vi "Scan Project Items.vi"(6 "Slide in":refnum<vi>, 7 "Project Path":path, 8 "error in (no error)":errorcluster, 10 "VI Refnum":refnum<vi>, 11 "Member Data in":string[][](array[string])) -> (0 "error out":errorcluster, 3 "Member Data out":string[][](array[string]))   [LabVIEW 2014]
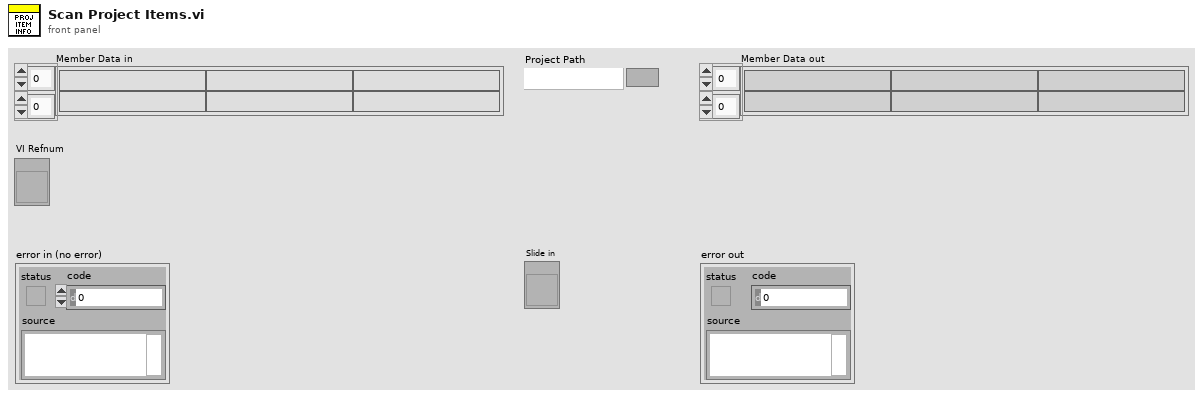
[diagram p1: front panel]
types:
  T1 = typedef "TYPE_Description Cluster.ctl" = cluster{"VI Description":string, "VI Version":string, "Review Date":string, "Author":string, "Copyright":string, "Requirements Coverage":string}
  T2 = typedef "TYPE_Version Status.ctl" = enum16{"Development", "alpha", "beta", "Reviewed", "Bug", "Other"}
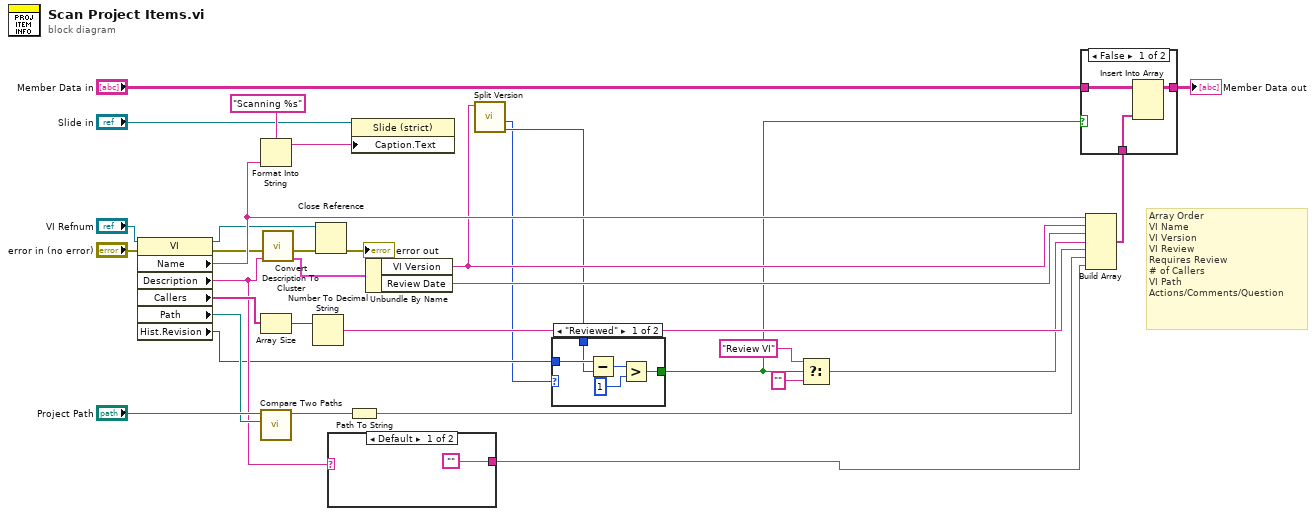
[diagram p0: block diagram]
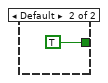
[diagram p2: hidden frame]
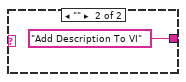
[diagram p3: hidden frame]
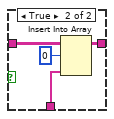
[diagram p4: hidden frame]
diagram:
  # "Array Order\nVI Name\nVI Version\nVI Review\nRequires Review\n# of Callers\nVI Path\nActions/Comments/Question"
  n1 = property class="VI"(reference="VI Refnum", error in="error in (no error)") -> (reference out=w9:refnum<vi>, error out=w14:errorcluster, "Name"=w23:string, "Description"=w13:string, "Callers"=w20:string[], "Path"=w18:path, "Hist.Revision"=w11:u32)
  n2 = Format Into String(format string="Scanning %s", w23) -> (resulting string=w27:string)  [unwired: 2 in, 1 out]
  n3 = Array Size(array=w20) -> (size(s)=w19:i32)
  n4 = call <vilib>:"Compare Two Paths.vi"("Path 2"=w18, "Path 1"="Project Path") -> ("Relative Path from 1 to 2"=w16:path)  [unwired: 6 in, 3 out]
  n5 = call <userlib>:"Convert Description To Cluster.vi"("Description String (empty)"=w13, "error in (no error)"=w14) -> ("Description Cluster"=w12:T1, "error out"=w8:errorcluster)  [unwired: 8 in]
  n6 = Number To Decimal String(number=w19) -> (decimal integer string=w17:string)  [unwired: 1 in]
  n7 = Close Reference(reference=w9, error in (no error)=w8) -> (error out=→"error out":errorcluster)
  n8 = case shown="Default" w13 {
    tunnel: ["" "Add Description To VI"] -> w6
    frame Default {
    }
    frame "" {
    }
  }
  n9 = Path To String(path=w16) -> (string=w22:string)
  n10 = property on="Property Node" class="Slide (strict)"(reference="Slide in", "Caption.Text"=w27) -> ()  [unwired: 1 in, 2 out]
  n11 = Unbundle By Name(w12) -> ("VI Version"=w15:string, "Review Date"=w21:string)
  n12 = call <userlib>:"Split Version.vi"("VI Version"=w15) -> ("Current Revision"=w10:u32, "Current Phase"=w1:T2)  [unwired: 7 in, 2 out]
  n13 = case shown="\"Reviewed\"" w1 {
    tunnel: w11 -> [w39 _]
    tunnel: w10 -> [w38 _]
    tunnel: [w35 TRUE] -> w5
    frame "Reviewed" {
      n14 = Subtract(x=w39, y=w38) -> (x-y=w37:u32)
      n15 = Greater?(x=w37, y=u32 1) -> (0:w35:bool)
    }
    frame Default {
    }
  }
  n16 = Select(t="Review VI", s=w5, f="") -> (s? t:f=w3:string)
  n17 = Build Array(w23, w15, w21, w3, w17, w22, w6) -> (w31:string[])
  n18 = case shown="False" w5 {
    tunnel: w31 -> [w43 w47]
    tunnel: "Member Data in" -> [w42 w46]
    tunnel: [w41 w45] -> w29
    frame False {
      n19 = Insert Into Array(array=w42, new element=w43) -> (w41:string[][])  [unwired: 2 in]
    }
    frame True {
      n20 = Insert Into Array(array=w46, index (row)=0, new element=w47) -> (w45:string[][])  [unwired: 1 in]
    }
  }
  "Member Data out" <- w29
